vi "Enum.vi"() -> ()   [LabVIEW 2019]
panel:
  in  "day":u8
  out "days_of_week 2":T1(ring)
  out "DayState":u8
  in  "days_of_week":T1(ring)
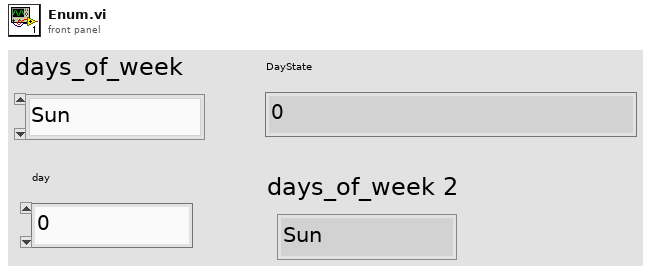
[diagram p1: front panel]
types:
  T1 = enum16{"Sun", "Mon", "Tue", "Wed", "Thurs", "Fri", "Sat"}
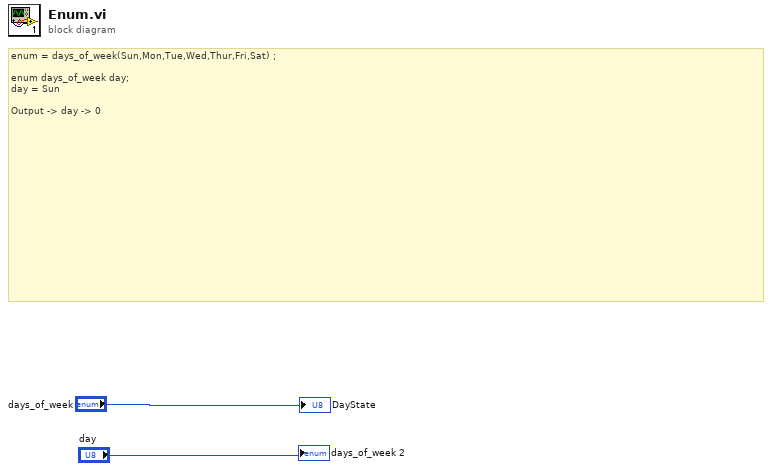
[diagram p0: block diagram]
diagram:
  # "enum = days_of_week(Sun,Mon,Tue,Wed,Thur,Fri,Sat) ;\n\nenum days_of_week day;\nday = Sun\n\nOutput -> day -> 0"
  "DayState" <- "days_of_week"
  "days_of_week 2" <- "day"
